vi "Histogram Main.vi"() -> ()   [LabVIEW 2012]
uses:
  Consumer Message.ctl
panel:
  out "Waveform Chart":dbl[](graph)
  in  "Snapshot":bool
  out "Histogram":cluster{"histogram":dbl[], "x axis":dbl[]}(graph)
  out "Consumer Shutdown?":bool
  in  "Stop":bool
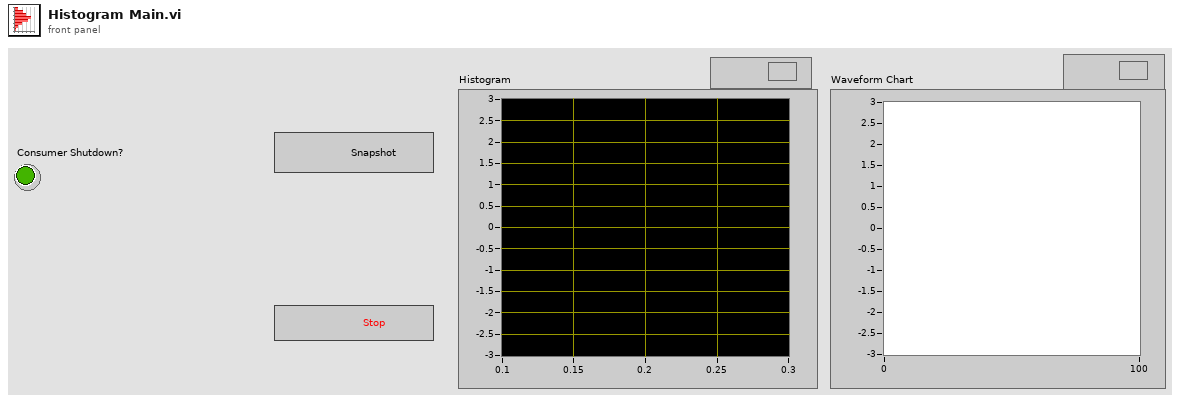
[diagram p1: front panel]
types:
  T1 = typedef "Consumer Message.ctl" = cluster{"Consumer State":string, "Boolean Data":bool, "Numeric Data":i32, "Signal":dbl[], "Error":errorcluster}
  T2 = enum32{"invalid app kind", "Development System", "Run Time System", "Student Edition", "Embedded LabVIEW", "Evaluation", "Custom"}
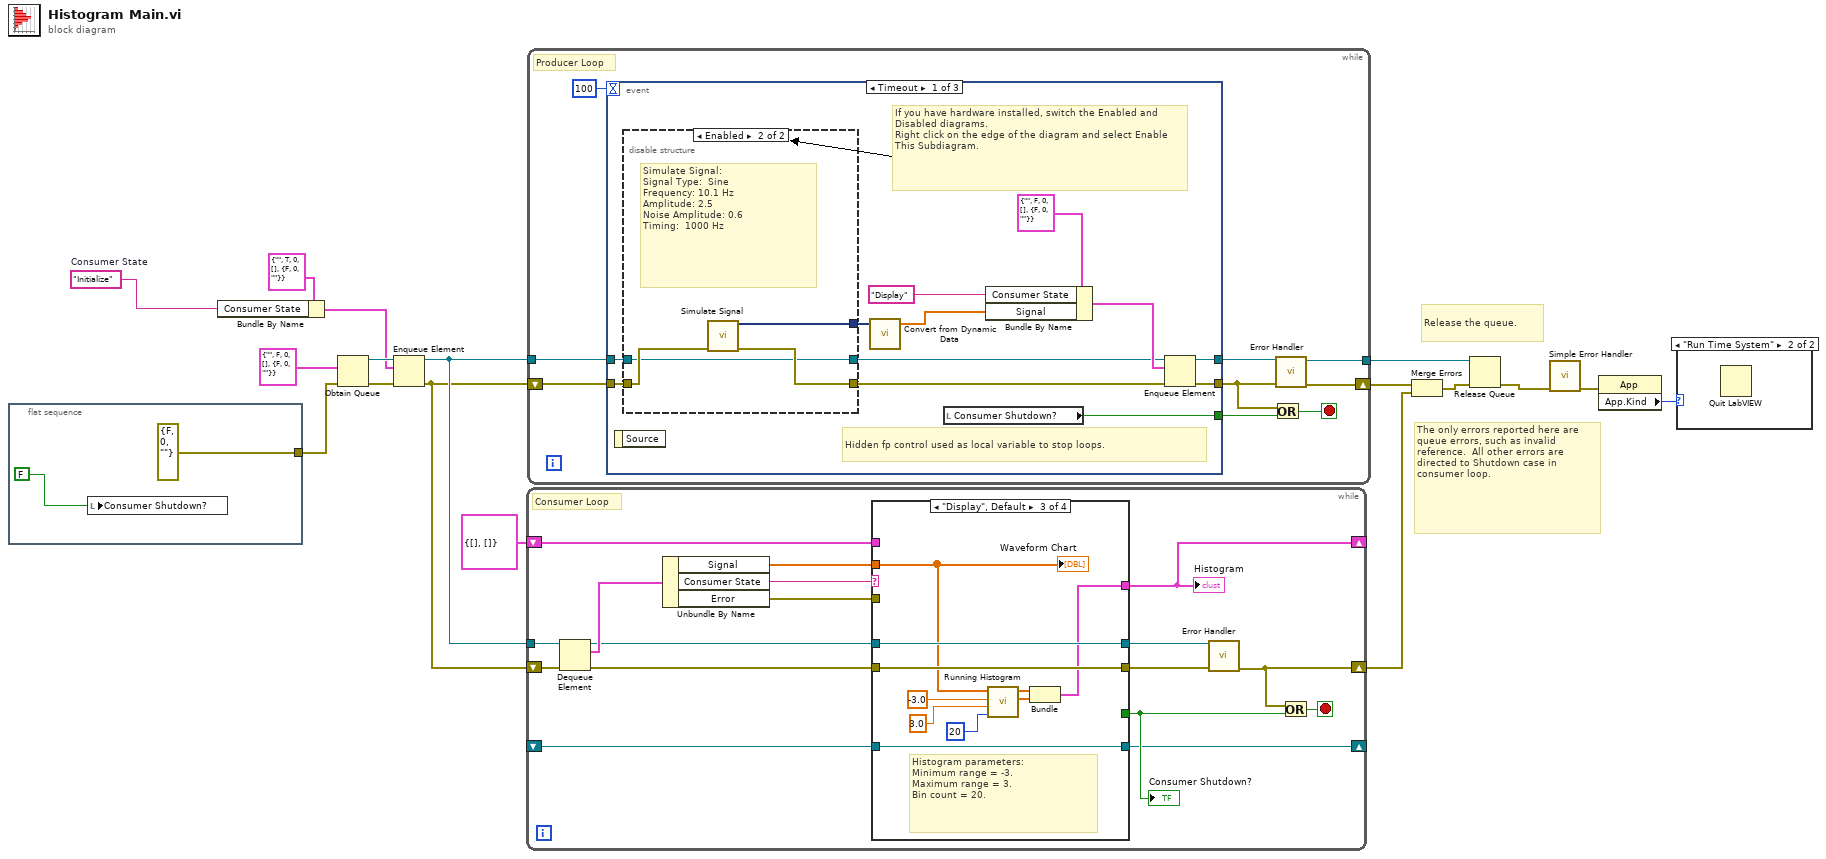
[diagram p0: block diagram]
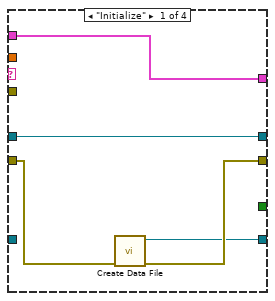
[diagram p3: hidden frame]
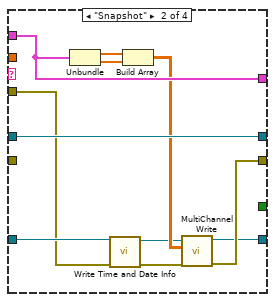
[diagram p4: hidden frame]
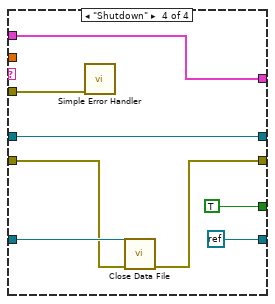
[diagram p5: hidden frame]
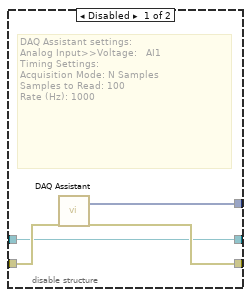
[diagram p6: hidden frame]
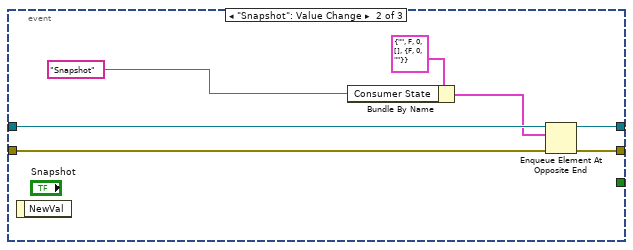
[diagram p7: hidden frame]
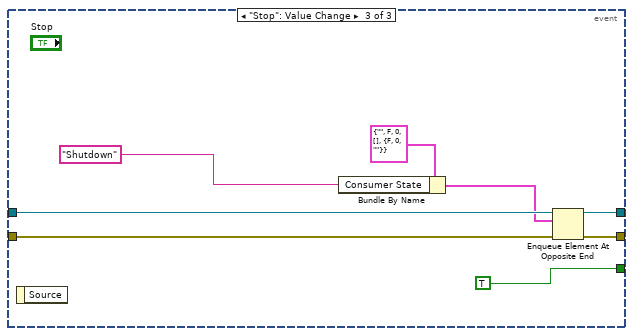
[diagram p8: hidden frame]
diagram:
  w10 = "Initialize"  # Consumer State
  # "Release the queue."
  # "The only errors reported here are queue errors, such as invalid reference.  All other errors are directed to Shutdown case in consumer loop."
  n1 = flat-sequence {
    tunnel: [errorcluster {"status"=FALSE, "code"=0, "source"=""} ("error in (no error)")] -> w13
    frame #0 {
      n2 = local write "Consumer Shutdown?"(FALSE ("Stop Loops (local)")) -> ()
    }
  }
  n3 = Bundle By Name(cluster=T1 {"Consumer State"="", "Boolean Data"=TRUE, "Numeric Data"=0, "Signal"=[], "Error"={"status"=FALSE, "code"=0, "source"=""}} ("Consumer Message"), "Consumer State"=w10) -> (w11:T1)
  n4 = Obtain Queue(element data type=T1 {"Consumer State"="", "Boolean Data"=FALSE, "Numeric Data"=0, "Signal"=[], "Error"={"status"=FALSE, "code"=0, "source"=""}}, error in (no error)=w13) -> (queue out=w15:refnum<queue>, error out=w17:errorcluster)  [unwired: 3 in, 1 out]
  n5 = Enqueue Element(queue=w15, element=w11, error in (no error)=w17) -> (queue out=w14:refnum<queue>, error out=w4:errorcluster)  [unwired: 1 in, 1 out]
  n6 = while {
    tunnel: w14 -> [w36]
    shift-right: [w27] -> w8
    shift-left: w4 -> [w35]
    shift-right: [w20] -> _
    shift-left: cluster{"histogram":dbl[], "x axis":dbl[]} {"histogram"=[], "x axis"=[]} -> [w24]
    shift-right: [w21] -> _
    shift-left: _ -> [w22]
    stop <- w28 stop-if-true
    # "Consumer Loop"
    n7 = Dequeue Element(queue=w36, error in (no error)=w35) -> (queue out=w26:refnum<queue>, element=w34:T1, error out=w25:errorcluster)  [unwired: 1 in, 1 out]
    n8 = Unbundle By Name(w34) -> ("Signal"=w23:dbl[], "Consumer State"=w33:string, "Error"=w30:errorcluster)
    n9 = case shown="\"Display\", Default" w33 {
      tunnel: [_ _ _ TRUE] -> w29
      tunnel: w25 -> [w39 _ w61 w65]
      tunnel: [w38 w48 w61 w64] -> w32
      tunnel: w26 -> [w41 w52 w62 w68]
      tunnel: [w41 w52 w62 w68] -> w31
      tunnel: w30 -> [_ w42 _ w69]
      tunnel: [w40 w50 w58 w67] -> w20
      tunnel: w24 -> [w40 w50 _ w67]
      tunnel: w23 -> [_ _ w56 _]
      tunnel: w22 -> [_ w43 w57 w66]
      tunnel: [w37 w47 w57 refnum<k0> refnum] -> w21
      frame "Initialize" {
        n10 = call "Create Data File.vi"("Error In"=w39) -> ("Error Out"=w38:errorcluster, "File Refnum"=w37:refnum<file>)  [unwired: 9 in]
      }
      frame "Snapshot" {
        n11 = Unbundle(w50) -> ("histogram"=w46:dbl[], "x axis"=w51:dbl[])
        n12 = call "Write Time and Date Info.vi"("Error In"=w42, "File Refnum In"=w43) -> ("Error Out"=w44:errorcluster, "File Refnum Out"=w45:refnum<file>)  [unwired: 6 in]
        n13 = Build Array(w46, w51) -> (w49:dbl[][])
        n14 = call "MultiChannel Write.vi"("Error In"=w44, "Data to Log"=w49, "File Refnum In"=w45) -> ("Error Out"=w48:errorcluster, "File Refnum Out"=w47:refnum<file>)  [unwired: 7 in]
      }
      frame "Display", Default {
        # "Histogram parameters:\nMinimum range = -3.\nMaximum range = 3. \nBin count = 20."
        n15 = call "Running Histogram.vi"("bins"=20, "max"=3.0, "min"=-3.0, "input data"=w56) -> ("x axis"=w59:dbl[], "histogram"=w60:dbl[])  [unwired: 4 in, 2 out]
        n16 = Bundle("histogram"=w60, "x axis"=w59) -> (w58:cluster{"histogram":dbl[], "x axis":dbl[]})  [unwired: 1 in]
        "Waveform Chart" <- w56
      }
      frame "Shutdown" {
        n17 = call <vilib>:"Simple Error Handler.vi"("error in (no error)"=w69) -> ()  [unwired: 4 in, 5 out]
        n18 = call "Close Data File.vi"("error in"=w65, "File Refnum In"=w66) -> ("error out"=w64:errorcluster)  [unwired: 9 in]
      }
    }
    "Consumer Shutdown?" <- w29
    "Histogram" <- w20
    n19 = call "Error Handler.vi"("error in"=w32, "queue in"=w31) -> ("error out"=w27:errorcluster)  [unwired: 8 in, 1 out]
    n20 = Or(x=w27, y=w29) -> (x .or. y?=w28:bool)
  }
  n21 = while {
    tunnel: w14 -> [w79]
    shift-right: [w72] -> w9
    shift-left: w4 -> [w78]
    tunnel: [w71] -> w3
    stop <- w74 stop-if-true
    # "Producer Loop"
    n22 = event shown="[0] Timeout" {
      selector: _ -> [_ _ _]
      dyn-events: _ -> [_ _ _]
      timeout: 100 -> [_ _ _]
      tunnel: w79 -> [w81 w105 w114]
      tunnel: w78 -> [w83 w104 w112]
      tunnel: [w86 w106 w111] -> w73
      tunnel: [w91 _ TRUE] -> w75
      tunnel: [w87 w101 w110] -> w77
      event Timeout {
        # "If you have hardware installed, switch the Enabled and Disabled diagrams.\nRight click on the edge of the diagram and select Enable This Subdiagram."
        # "Hidden fp control used as local variable to stop loops."
        n23 = event-data() -> ()  [unwired: 1 in, 1 out]
        n24 = disable-structure shown="Enabled" {
          disable-tunnel: [w95 w97] -> w84
          disable-tunnel: w83 -> [w94 w99]
          disable-tunnel: [w93 w98] -> w82
          disable-tunnel: w81 -> [w92 w96]
          disable-tunnel: [w92 w96] -> w80
          frame Disabled {
            # "DAQ Assistant settings:\nAnalog Input>>Voltage:   AI1\nTiming Settings:\nAcquisition Mode: N Samples\nSamples to Read: 100\nRate (Hz): 1000"
            n25 = call "DAQ Assistant"("error in"=w94) -> ("data"=w95:dynamicdata, "error out"=w93:errorcluster)  [unwired: 16 in, 1 out]
          }
          frame Enabled {
            # "Simulate Signal:\nSignal Type:  Sine\nFrequency: 10.1 Hz\nAmplitude: 2.5\nNoise Amplitude: 0.6\nTiming:  1000 Hz"
            n26 = call "Simulate Signal"("error in (no error)"=w99) -> ("Sine with Uniform Noise"=w97:dynamicdata, "error out"=w98:errorcluster)  [unwired: 13 in]
          }
        }
        n27 = call "Convert from Dynamic Data"("Dynamic Data Type"=w84) -> ("Array"=w85:dbl[])  [unwired: 3 in]
        n28 = local read "Consumer Shutdown?"() -> (w91:bool)
        n29 = Bundle By Name(cluster=T1 {"Consumer State"="", "Boolean Data"=FALSE, "Numeric Data"=0, "Signal"=[], "Error"={"status"=FALSE, "code"=0, "source"=""}}, "Consumer State"="Display", "Signal"=w85) -> (w89:T1)
        n30 = Enqueue Element(queue=w80, element=w89, error in (no error)=w82) -> (queue out=w87:refnum<queue>, error out=w86:errorcluster)  [unwired: 1 in, 1 out]
      }
      event "Snapshot": Value Change {
        n31 = event-data() -> ()  [unwired: 1 in, 1 out]
        n32 = Bundle By Name(cluster=T1 {"Consumer State"="", "Boolean Data"=FALSE, "Numeric Data"=0, "Signal"=[], "Error"={"status"=FALSE, "code"=0, "source"=""}}, "Consumer State"="Snapshot" ("String Data")) -> (w102:T1)
        n33 = Enqueue Element At Opposite End(queue=w105, element=w102, error in (no error)=w104) -> (queue out=w101:refnum<queue>, error out=w106:errorcluster)  [unwired: 1 in, 1 out]
      }
      event "Stop": Value Change {
        n34 = event-data() -> ()  [unwired: 1 in, 1 out]
        n35 = Bundle By Name(cluster=T1 {"Consumer State"="", "Boolean Data"=FALSE, "Numeric Data"=0, "Signal"=[], "Error"={"status"=FALSE, "code"=0, "source"=""}}, "Consumer State"="Shutdown") -> (w107:T1)
        n36 = Enqueue Element At Opposite End(queue=w114, element=w107, error in (no error)=w112) -> (queue out=w110:refnum<queue>, error out=w111:errorcluster)  [unwired: 1 in, 1 out]
      }
    }
    n37 = Or(x=w73, y=w75) -> (x .or. y?=w74:bool)
    n38 = call "Error Handler.vi"("error in"=w73, "queue in"=w77) -> ("error out"=w72:errorcluster, "queue out"=w71:refnum<queue>)  [unwired: 8 in]
  }
  n39 = Merge Errors(w9, w8) -> (w6:errorcluster)
  n40 = Release Queue(queue=w3, error in (no error)=w6) -> (error out=w5:errorcluster)  [unwired: 1 in, 2 out]
  n41 = call <vilib>:"Simple Error Handler.vi"("error in (no error)"=w5) -> ("error out"=w1:errorcluster)  [unwired: 4 in, 4 out]
  n42 = property class="App"(error in=w1) -> ("App.Kind"=w2:T2)  [unwired: 1 in, 2 out]
  n43 = case shown="\"Run Time System\"" w2 {
    frame "invalid app kind", Default {
    }
    frame "Run Time System" {
      n44 = Quit LabVIEW() -> ()  [unwired: 1 in]
    }
  }
